vi "FIRE_ATMEGA_LABVIEW_RXTX.vi"() -> ()   [LabVIEW 2013]
uses:
  D:/Program Files (x86)/National Instruments/LabVIEW 2013/examples/Instrument IO/Serial/support/Serial - Settings.ctl
  <vilib>/Instr/_visa.llb/VISA Configure Serial Port (Instr).vi
panel:
  out "?":bool
  out "?":bool
  out "NO MOTION DETECTED":bool
  out "MOTION DETECTED":bool
  in  "stop":bool
  out "Waveform Chart":i32(graph)
  out "MOTION LEVEL VARIABLE":string
  out "read buffer":string
  in  "byte count":u32
  in  "Serial Settings":T1={"baud rate"=9600, "data bits"=8, "parity"=enum."None", "stop bits"=10, "flow control"=0} {"flow control" items=["None"=0, "XON/XOFF"=1, "RTS/CTS"=2, "DTR/DSR"=4]; "stop bits" items=["1.0"=10, "1.5"=15, "2.0"=20]; "data bits" min=5 max=8 step=1; "baud rate" items=["75"=75, "110"=110, "134"=134, "150"=150, "300"=300, "600"=600, "1200"=1200, "1800"=1800, "2400"=2400, "4800"=4800, "7200"=7200, "9600"=9600, "14400"=14400, "19200"=19200, "28800"=28800, "38400"=38400, "56000"=56000, "57600"=57600, "115200"=115200, "128000"=128000, "230400"=230400]}
  in  "VISA resource name":refnum<visa-resource-name>
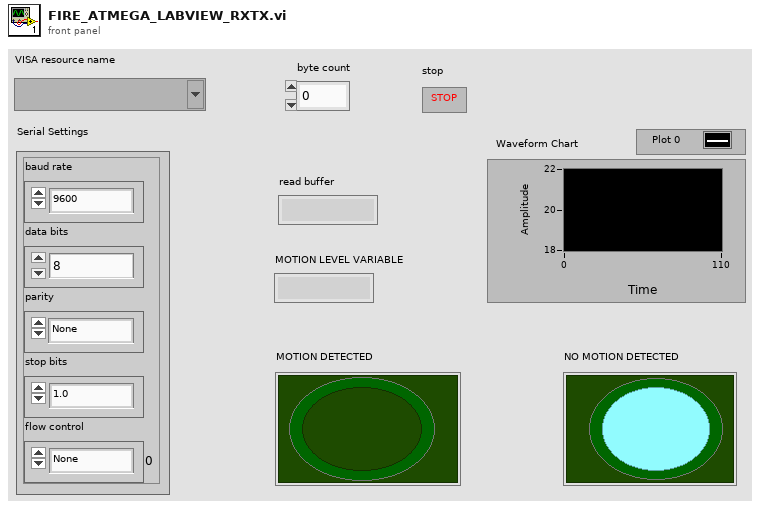
[diagram p1: front panel]
types:
  T1 = typedef "Serial - Settings.ctl" = cluster{"baud rate":u32, "data bits":u16, "parity":enum16{"None", "Odd", "Even", "Mark", "Space"}, "stop bits":u16, "flow control":u16}
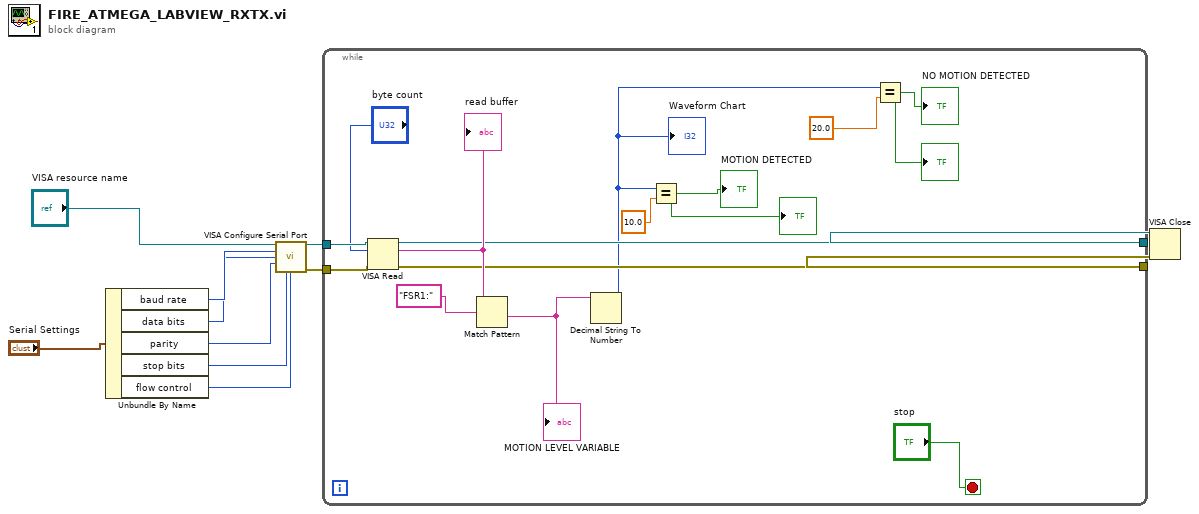
[diagram p0: block diagram]
diagram:
  n1 = Unbundle By Name("Serial Settings") -> ("baud rate"=w9:u32, "data bits"=w8:u16, "parity"=w7:enum16{"None", "Odd", "Even", "Mark", "Space"}, "stop bits"=w6:u16, "flow control"=w5:u16)
  n2 = call-poly "VISA Configure Serial Port"("VISA resource name"="VISA resource name", "baud rate (9600)"=w9, "data bits (8)"=w8, "parity (0:none)"=w7, "stop bits (10: 1 bit)"=w6, "flow control (0:none)"=w5) -> ("VISA resource name out"=w4:refnum<visa-resource-name>, "error out"=w3:errorcluster)  [unwired: 8 in]
  n3 = while {
    tunnel: w4 -> [w25]
    tunnel: w3 -> [w24]
    tunnel: [w20] -> w2
    tunnel: [w19] -> w1
    stop <- "stop" stop-if-true
    n4 = VISA Read(VISA resource name=w25, byte count="byte count", error in (no error)=w24) -> (VISA resource name out=w19:refnum<visa-resource-name>, read buffer=w22:string, error out=w20:errorcluster)  [unwired: 1 out]
    "read buffer" <- w22
    n5 = Match Pattern(string=w22, regular expression="FSR1:") -> (after substring=w15:string)  [unwired: 1 in, 3 out]
    "MOTION LEVEL VARIABLE" <- w15
    n6 = Decimal String To Number(string=w15) -> (number=w14:i32)  [unwired: 2 in, 1 out]
    "Waveform Chart" <- w14
    n7 = Equal?(x=w14, y=10.0) -> (x = y?=→"MOTION DETECTED" →"?":bool)
    n8 = Equal?(x=w14, y=20.0) -> (x = y?=→"NO MOTION DETECTED" →"?":bool)
  }
  n9 = VISA Close(VISA resource name=w1, error in (no error)=w2) -> ()  [unwired: 1 out]
